vi "Create Response-JSONtext.vi"(6 "id":string, 8 "error in (no error)":errorcluster, 10 "result":variant) -> (0 "error out":errorcluster, 2 "{JSON}":string)   [LabVIEW 2019, in "JSON-RPC.lvclass"]
uses:
  JSON-RPC.lvclass
  31d5db40-9dcb-43d1-a6f6-9a2e0a5d4432.vi
  c6edfa98-d038-4790-952c-164baa6befaa.vi
  8b9e59fa-9ebd-4504-a939-6047597c77d3.vi
  <vilib>/JDP Science/JSONtext/Variant to JSON Text.vi
  <vilib>/JDP Science/JSONtext/LVClass Serializer/JSONtext LVClass Serializer.lvclass
  <vilib>/JDP Science/JSONtext/JSONtext.lvlib
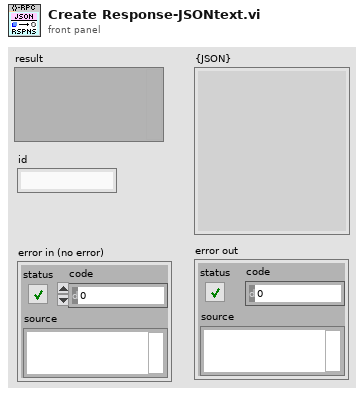
[diagram p1: front panel]
types:
  T1 = cluster{"jsonrpc":string, "result":string, "id":string}
  T2 = typedef "JSON-RPC.lvclass/Error--Cluster.ctl" = cluster{"code":i32, "message":string}
  T3 = cluster{"jsonrpc":string, "error":T2, "id":string}
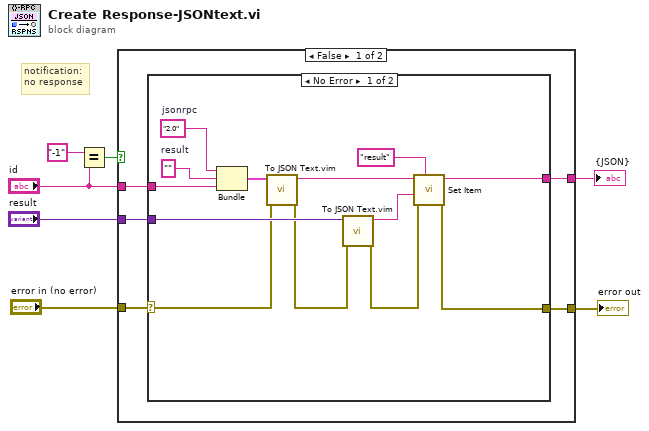
[diagram p0: block diagram]
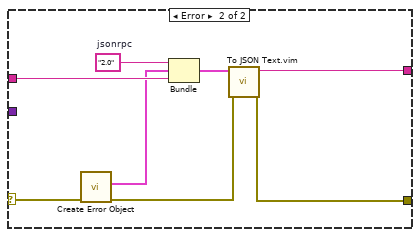
[diagram p2: hidden frame]
diagram:
  # "notification:\nno response"
  n1 = Equal?(x="-1", y="id") -> (x = y?=w1:bool)
  n2 = case shown="False" w1 {
    tunnel: [w12 w34] -> w7
    tunnel: [w11 _] -> w6
    tunnel: "result" -> [w10 _]
    tunnel: "error in (no error)" -> [w9 w34]
    tunnel: "id" -> [w8 _]
    frame False {
      n3 = case shown="No Error" w9 {
        selector: w9 -> [w21 w28]
        tunnel: [w13 w32] -> w12
        tunnel: [w20 w33] -> w11
        tunnel: w8 -> [w15 w31]
        tunnel: w10 -> [w25 _]
        frame No Error {
          w14 = ""  # result
          w17 = "2.0"  # jsonrpc
          n4 = Bundle("jsonrpc"=w17, "result"=w14, "id"=w15) -> (w16:T1)  [unwired: 1 in]
          n5 = call "To JSON Text.vim"("error in (no error)"=w21, "Anything"=w16) -> ("error out"=w19:errorcluster, "<JSON>"=w18:string)  [unwired: 8 in]
          n6 = call "To JSON Text.vim"("error in (no error)"=w19, "Anything"=w25) -> ("error out"=w24:errorcluster, "<JSON>"=w23:string)  [unwired: 8 in]
          n7 = call <vilib>:"Set Item.vi"("$Path or Item Name"="result", "error in (no error)"=w24, "JSON to Insert"=w23, "JSON"=w18) -> ("error out"=w13:errorcluster, "<JSON>"=w20:string)  [unwired: 4 in, 1 out]
        }
        frame Error {
          w29 = "2.0"  # jsonrpc
          n8 = call "Create Error Object.vi"("error in (no error)"=w28) -> ("error out"=w27:errorcluster, "error"=w26:T2)  [unwired: 9 in]
          n9 = Bundle("jsonrpc"=w29, "error"=w26, "id"=w31) -> (w30:T3)  [unwired: 1 in]
          n10 = call "To JSON Text.vim"("error in (no error)"=w27, "Anything"=w30) -> ("error out"=w32:errorcluster, "<JSON>"=w33:string)  [unwired: 8 in]
        }
      }
    }
    frame True {
    }
  }
  "error out" <- w7
  "{JSON}" <- w6
